vi "write laser line.vi"(8 "error in (no error)":errorcluster, 11 "AOTF in":refnum<class "AOTF.lvclass">) -> (0 "error out":errorcluster, 3 "AOTF out":refnum<class "AOTF.lvclass">)   [LabVIEW 2012, in "AOTF.lvclass"]
uses:
  AOTF.lvclass
panel:
  out "concatenated string":string
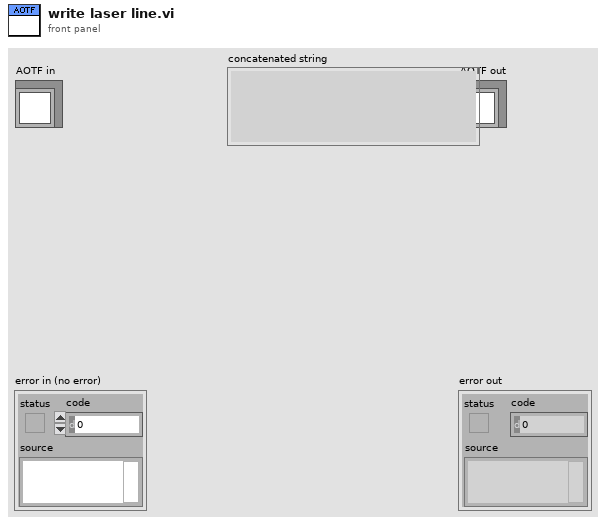
[diagram p1: front panel]
types:
  T1 = typedef "AOTF.lvclass/laser line enum.ctl" = dbl
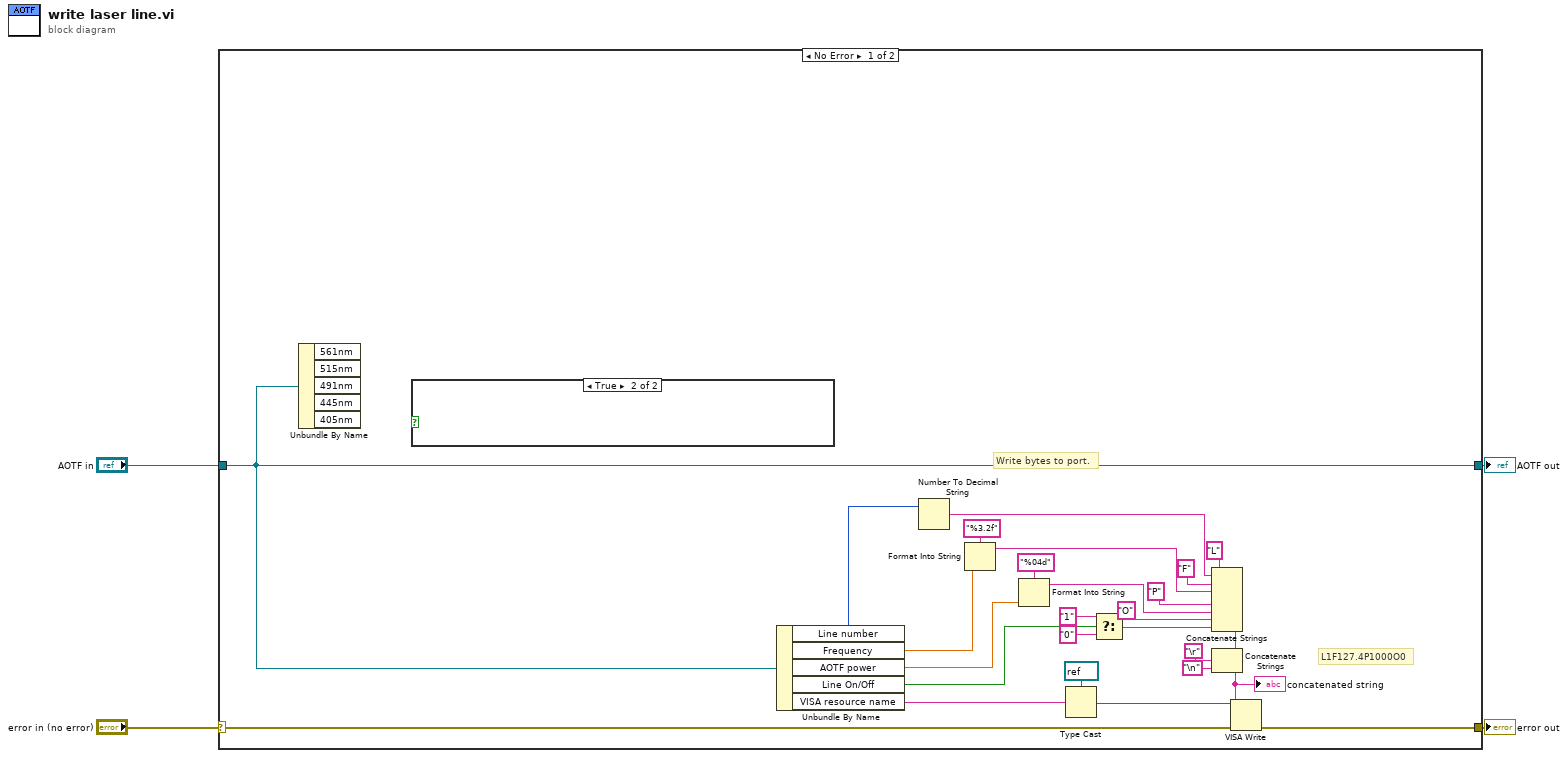
[diagram p0: block diagram]
diagram:
  n1 = case shown="No Error" "error in (no error)" {
    selector: "error in (no error)" -> [w6 w32]
    tunnel: [w7 w32] -> w3
    tunnel: [w5 w31] -> w1
    tunnel: "AOTF in" -> [w5 w31]
    frame No Error {
      # "L1F127.4P1000O0"
      # "Write bytes to port."
      n2 = Unbundle By Name(w5) -> ()  [unwired: 5 out]
      n3 = case shown="True" {
        selector: _ -> [_ _]
        frame False {
        }
        frame True {
        }
      }
      n4 = Unbundle By Name(w5) -> ("Line number"=w19:u32, "Frequency"=w21:T1, "AOTF power"=w24:dbl, "Line On/Off"=w30:bool, "VISA resource name"=w16:string)
      n5 = Number To Decimal String(number=w19) -> (decimal integer string=w18:string)  [unwired: 1 in]
      n6 = Format Into String(format string="%3.2f", w21) -> (resulting string=w23:string)  [unwired: 2 in, 1 out]
      n7 = Format Into String(format string="%04d", w24) -> (resulting string=w25:string)  [unwired: 2 in, 1 out]
      n8 = Type Cast(type=refnum<visa-resource-name> refnum ("VISA resource name"), x=w16) -> (*(type *) &x=w20:refnum<visa-resource-name>)
      n9 = Select(t="1" ("string"), s=w30, f="0" ("string")) -> (s? t:f=w27:string)
      n10 = Concatenate Strings("L", w18, "F" ("string"), w23, "P" ("string"), w25, "O" ("string"), w27) -> (w8:string)
      n11 = Concatenate Strings(w8, "\r", "\n") -> (w14:string)
      "concatenated string" <- w14
      n12 = VISA Write(VISA resource name=w20, write buffer=w14, error in (no error)=w6) -> (error out=w7:errorcluster)  [unwired: 2 out]
    }
    frame Error {
    }
  }
  "error out" <- w3
  "AOTF out" <- w1
